vi "add scan current(SubVI).vi"(10 "字符串":string) -> (1 "ok or cancel":bool=TRUE, 2 "连接的字符串":string)   [LabVIEW 2019, in "Add Seq.lvlib"]
uses:
  Add Seq.lvlib
panel:
  in  "Number of Step":i32=2
  in  "Increments (mA)":dbl=10.0
  in  "Final Current (mA)":dbl
  in  "Initial Current(mA)":dbl
  in  "cancel":bool
  in  "ok":bool
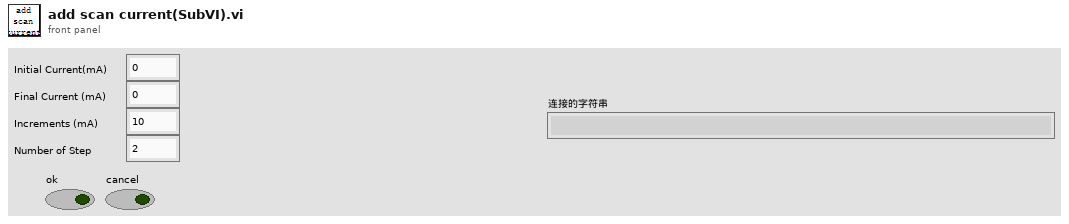
[diagram p1: front panel]
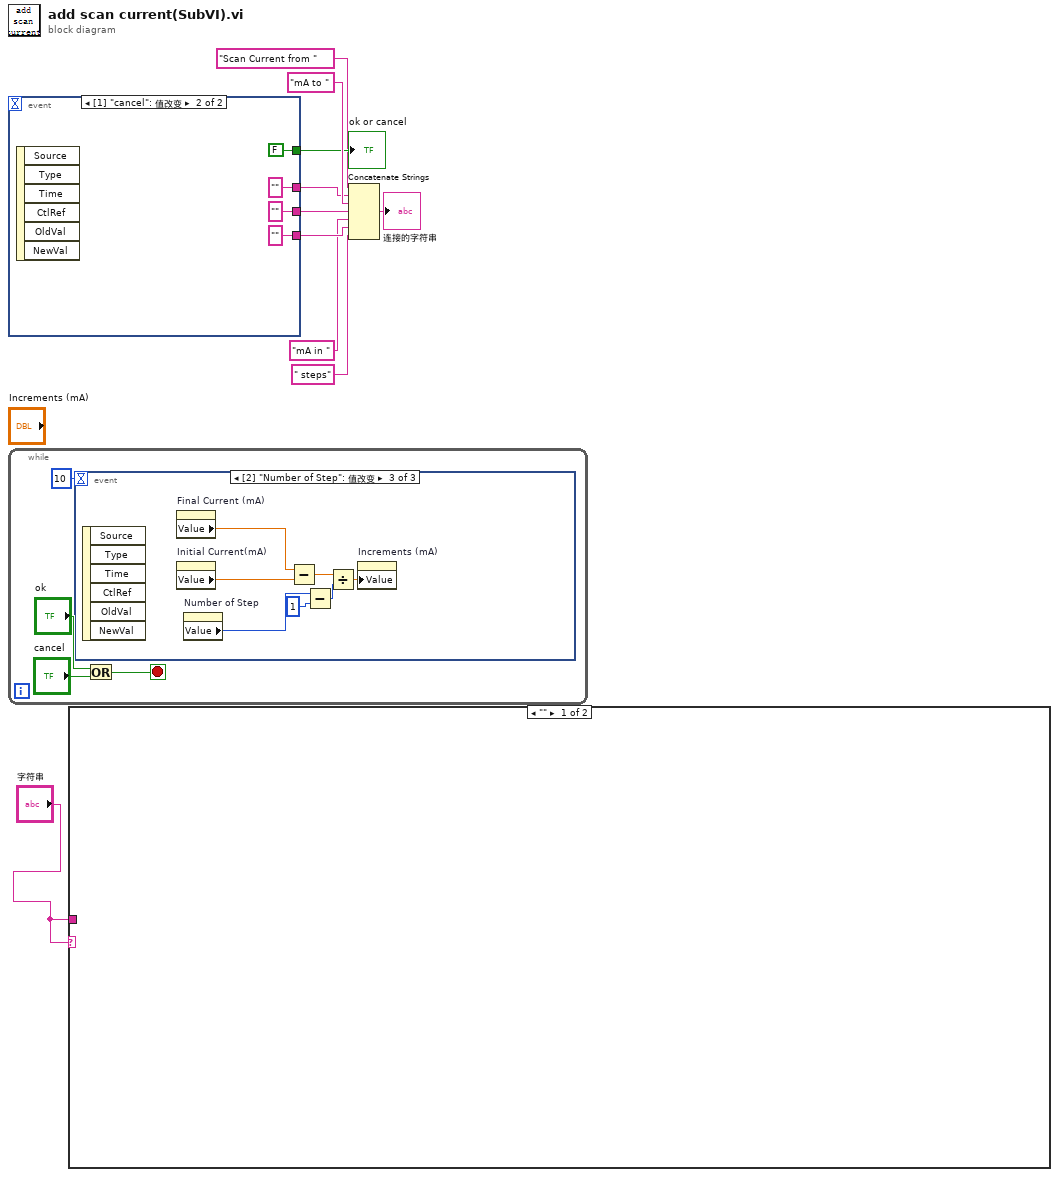
[diagram p0: block diagram]
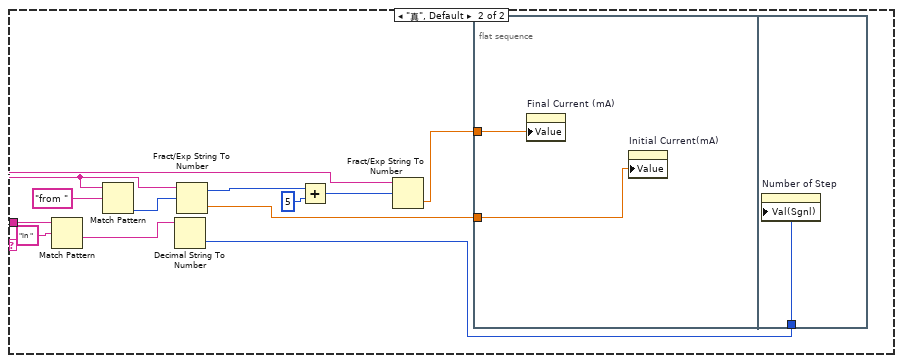
[diagram p2: hidden frame]
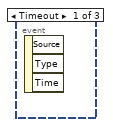
[diagram p3: hidden frame]
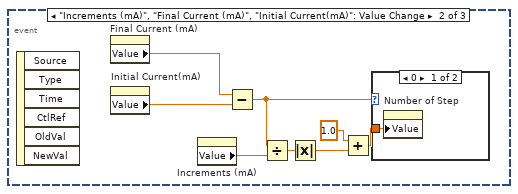
[diagram p4: hidden frame]
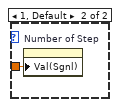
[diagram p5: hidden frame]
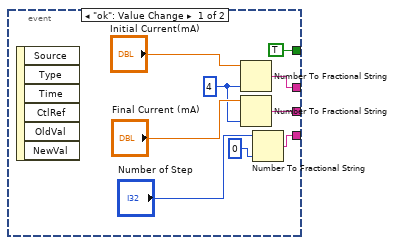
[diagram p6: hidden frame]
diagram:
  n1 = event shown="[1] \"cancel\": 值改变" {
    selector: _ -> [_ _]
    dyn-events: _ -> [_ _]
    timeout: _ -> [_ _]
    tunnel: [TRUE FALSE] -> w8
    tunnel: [w17 ""] -> w6
    tunnel: [w15 ""] -> w4
    tunnel: [w12 ""] -> w3
    event "ok": Value Change {
      w13 = i16 4 ("精度(6)")
      n2 = event-data() -> ()  [unwired: 1 in, 6 out]
      n3 = Number To Fractional String(number="Initial Current(mA)", precision (6)=w13) -> (F-format string=w17:string)  [unwired: 2 in]
      n4 = Number To Fractional String(number="Final Current (mA)", precision (6)=w13) -> (F-format string=w12:string)  [unwired: 2 in]
      n5 = Number To Fractional String(number="Number of Step", precision (6)=i16 0 ("精度(6)")) -> (F-format string=w15:string)  [unwired: 2 in]
    }
    event "cancel": Value Change {
      n6 = event-data() -> ()  [unwired: 1 in, 6 out]
    }
  }
  "ok or cancel" <- w8
  n7 = while {
    stop <- w26 stop-if-true
    n8 = event shown="[2] \"Number of Step\": 值改变" {
      selector: _ -> [_ _ _]
      dyn-events: _ -> [_ _ _]
      timeout: 10 -> [_ _ _]
      event Timeout {
        n9 = event-data() -> ()  [unwired: 1 in, 3 out]
      }
      event "Increments (mA)", "Final Current (mA)", "Initial Current(mA)": Value Change {
        n10 = event-data() -> ()  [unwired: 1 in, 6 out]
        n11 = property on="Final Current (mA)" class="DigNum (严格)"() -> ("Value"=w32:dbl)  [unwired: 2 in, 2 out]
        n12 = property on="Initial Current(mA)" class="DigNum (严格)"() -> ("Value"=w31:dbl)  [unwired: 2 in, 2 out]
        n13 = property on="Increments (mA)" class="DigNum (严格)"() -> ("Value"=w30:dbl)  [unwired: 2 in, 2 out]
        n14 = Subtract(x=w32, y=w31) -> (x-y=w28:dbl)
        n15 = Divide(x=w28, y=w30) -> (x/y=w34:dbl)
        n16 = Absolute Value(x=w34) -> (abs(x)=w33:dbl)
        n17 = Add(x=1.0, y=w33) -> (x+y=w29:dbl)
        n18 = case shown="0" w28 {
          tunnel: w29 -> [w36 w37]
          frame 0 {
            n19 = property on="Number of Step" class="DigNum (严格)"("Value"=w36) -> ()  [unwired: 2 in, 2 out]
          }
          frame 1, Default {
            n20 = property on="Number of Step" class="DigNum (严格)"("Val(Sgnl)"=w37) -> ()  [unwired: 2 in, 2 out]
          }
        }
      }
      event "Number of Step": Value Change {
        n21 = event-data() -> ()  [unwired: 1 in, 6 out]
        n22 = property on="Final Current (mA)" class="DigNum (严格)"() -> ("Value"=w41:dbl)  [unwired: 2 in, 2 out]
        n23 = property on="Initial Current(mA)" class="DigNum (严格)"() -> ("Value"=w40:dbl)  [unwired: 2 in, 2 out]
        n24 = property on="Number of Step" class="DigNum (严格)"() -> ("Value"=w39:i32)  [unwired: 2 in, 2 out]
        n25 = Subtract(x=w41, y=w40) -> (x-y=w44:dbl)
        n26 = Subtract(x=w39, y=1) -> (x-y=w42:i32)
        n27 = Divide(x=w44, y=w42) -> (x/y=w38:dbl)
        n28 = property on="Increments (mA)" class="DigNum (严格)"("Value"=w38) -> ()  [unwired: 2 in, 2 out]
      }
    }
    n29 = Or(x="ok", y="cancel") -> (x .or. y?=w26:bool)
  }
  n30 = case shown="\"\"" "字符串" {
    tunnel: "字符串" -> [_ w48]
    frame "" {
    }
    frame "真", Default {
      n31 = Match Pattern(string=w48, regular expression="in " ("正则表达式")) -> (after substring=w49:string)  [unwired: 1 in, 3 out]
      n32 = Match Pattern(string=w48, regular expression="from " ("正则表达式")) -> (offset past match=w53:i32)  [unwired: 1 in, 3 out]
      n33 = Decimal String To Number(string=w49) -> (number=w45:i32)  [unwired: 2 in, 1 out]
      n34 = Fract/Exp String To Number(string=w48, offset=w53) -> (offset past number=w51:i32, number=w47:dbl)  [unwired: 2 in]
      n35 = Add(x=w51, y=5) -> (x+y=w52:i32)
      n36 = Fract/Exp String To Number(string=w48, offset=w52) -> (number=w46:dbl)  [unwired: 2 in, 1 out]
      n37 = flat-sequence {
        tunnel: w47 -> [w57]
        tunnel: w46 -> [w56]
        tunnel: w45 -> [w58]
        frame #0 {
          n38 = property on="Final Current (mA)" class="DigNum (严格)"("Value"=w56) -> ()  [unwired: 2 in, 2 out]
          n39 = property on="Initial Current(mA)" class="DigNum (严格)"("Value"=w57) -> ()  [unwired: 2 in, 2 out]
        }
        frame #1 {
          n40 = property on="Number of Step" class="DigNum (严格)"("Val(Sgnl)"=w58) -> ()  [unwired: 2 in, 2 out]
        }
      }
    }
  }
  n41 = Concatenate Strings("Scan Current from " ("字符串"), w6, "mA to " ("字符串"), w3, "mA in " ("字符串"), w4, " steps" ("字符串")) -> (→"连接的字符串":string)
